vi "User Interface.vi"(10 "Test File Path":path=path "") -> ()   [LabVIEW 2020, in "Execution UI.lvclass"]
uses:
  Execution UI.lvclass
  Execution UI.lvclass/Execution UI.ctl
  Process/Process.lvclass
  <vilib>/Utility/miscctls.llb/LVNodeAndColumnTypeDef.ctl
  Private/TypeDefs/Execution State.ctl
  <vilib>/Platform/browser.llb/Open URL in Default Browser (string).vi
  Core/Result/Status.ctl
  Core/Result/Result.lvlib
  Result Model by Reference/Result Model by Reference.lvclass
  Core/Result/Type.ctl
  Core/Result/Result.ctl
  Configuration Manager/Configuration Manager.lvclass
  Support/Utilities.lvlib
  Error Handler/Error Handler.lvclass
  Framework/Test Finder/Test Finder.lvclass
  Framework/Test Runner/Test Runner.lvclass
  Result Model/Tree Item Filter.ctl
  Result Model/Result Model.lvclass
  Framework/Plugin/Plugin.lvclass
  C:/git/astemes-lunit/source/User Interface/Process/Process.lvclass
  C:/git/astemes-lunit/source/User Interface/Execution UI/Execution UI.lvclass
  C:/git/astemes-lunit/source/Framework/Result Observer/Result Observer.lvclass
panel:
  in  "Refresh":bool
  in  "Run Selected Tests":bool
  in  "Stop":bool
  in  "Run All Tests":bool
  in  "Eject":bool
  in  "Collapse":bool
  in  "Expand":bool
  out "Progress bar":dbl(slide) scale=0.0..100.0
  out "Results":i32(listbox)=-1
  in  "Test Results":string[](tree)
  out "Shift?":bool
  in  "Filter fails":bool
  out "Description":string
  out "Status":string
  # "1"
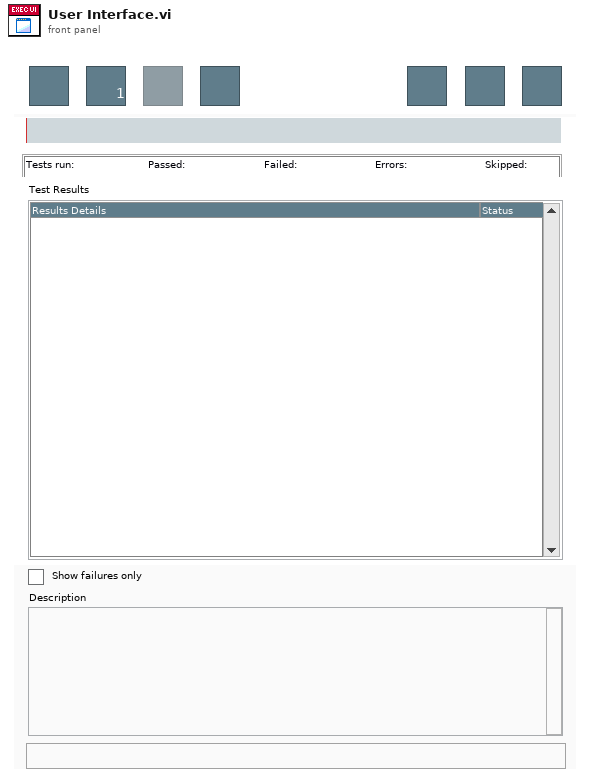
[diagram p1: front panel]
types:
  T1 = typedef "Execution UI.lvclass/Execution State.ctl" = enum16{"Idle", "Running"}
  T2 = typedef "Result.lvlib/Result.ctl" = cluster{"Name":string, "Message":string, "Description":string, "Status":T3, "Result Type":T4, "Execution Time":dbl}
  T3 = typedef "Result.lvlib/Status.ctl" = enum16{"", "Passed", "Failed", "Error", "Skipped", "Setup Error", "Broken", "Teardown Error"}
  T4 = typedef "Result.lvlib/Type.ctl" = enum16{"Test Case", "Test Suite", "Test Run", "Pass", "Fail", "Skip", "Pass if", "Fail if", "Pass if Error", "Fail if Error", "Pass if Equal", "Fail if Equal"}
  T5 = typedef "LVNodeAndColumnTypeDef.ctl" = cluster{"Node":string, "Column":i32}
  T6 = enum8{"Enabled", "Disabled", "Disabled and Grayed Out"}
  T7 = typedef "Result Model.lvclass/Tree Item Filter.ctl" = enum16{"All", "Only Fails", "Fails or else Not Executed"}
  T8 = enum32{"Invalid", "Standard", "Closed", "Hidden", "Minimized", "Maximized"}
  T9 = typedef "Result Model.lvclass/Statistics.ctl" = cluster{"Method Count":u32, "Executed Methods":u32, "Passed Methods":u32, "Failed Methods":u32, "Method Errors":u32, "Skipped Method":u32, "Progress [%]":dbl}
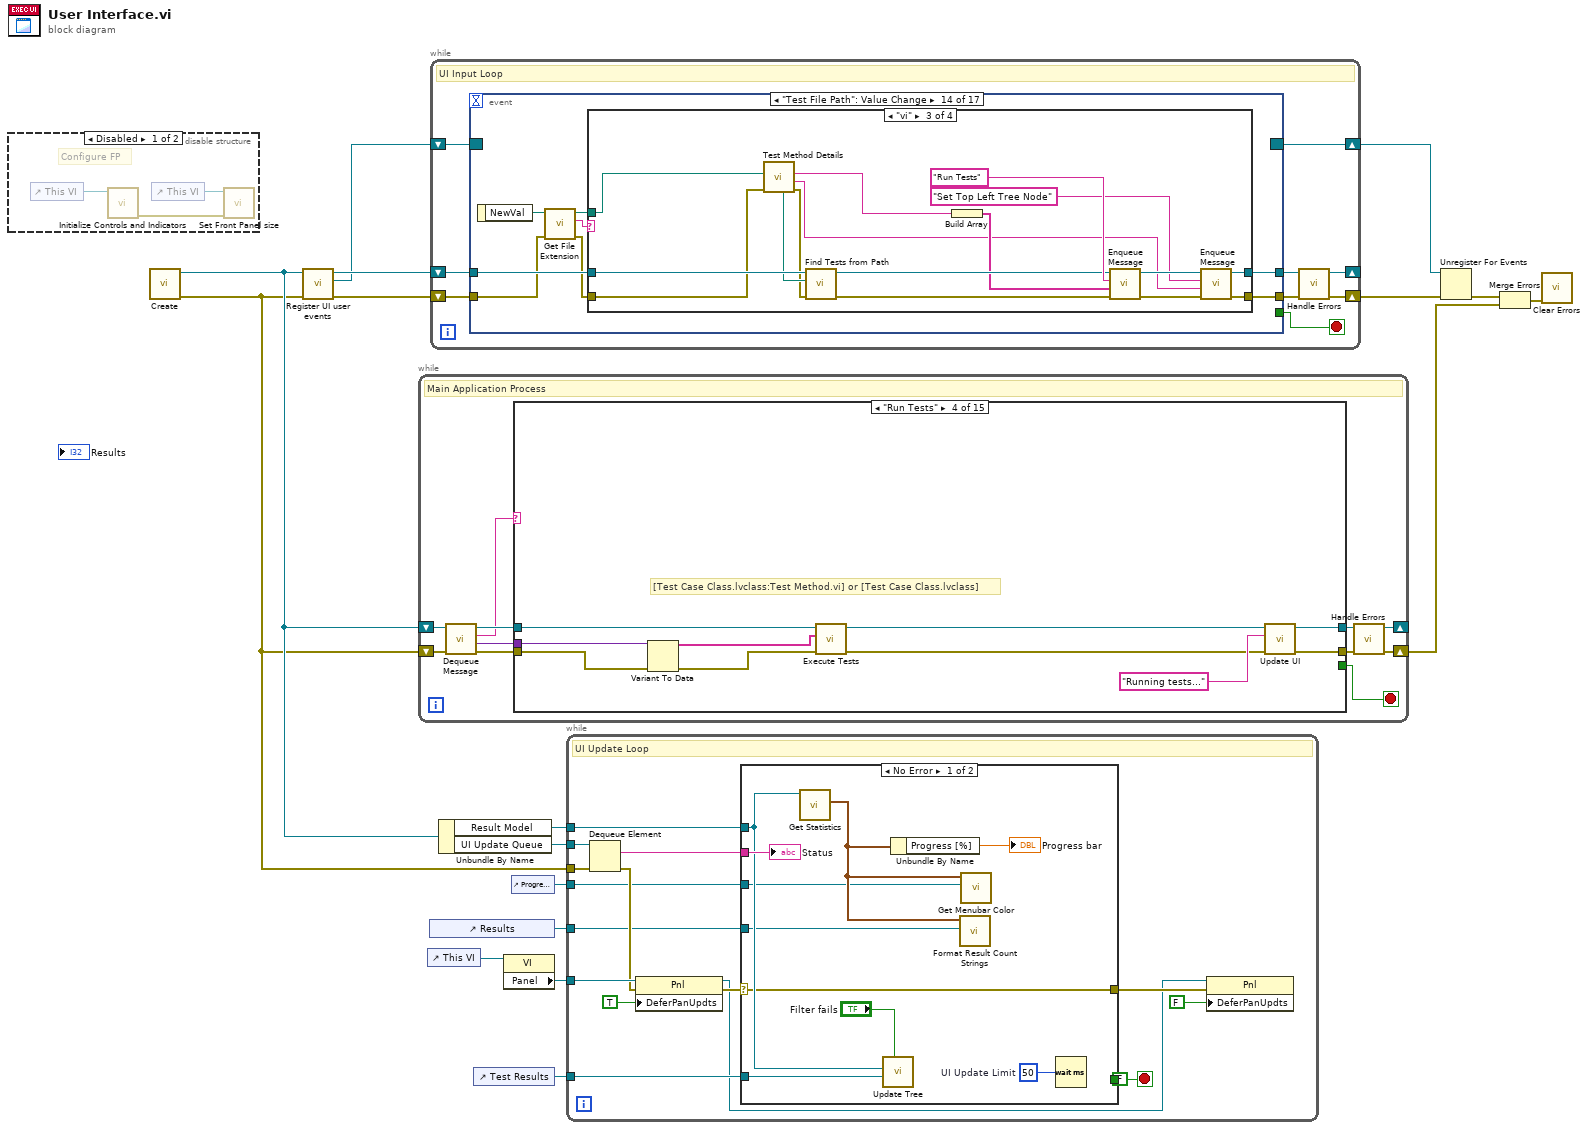
[diagram p0: block diagram]
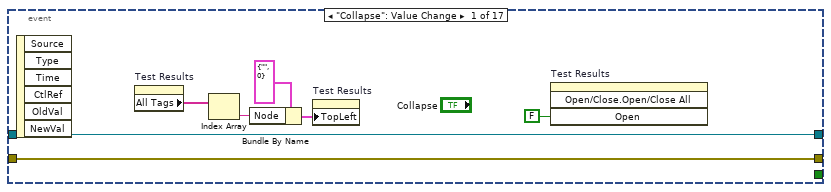
[diagram p2: hidden frame]
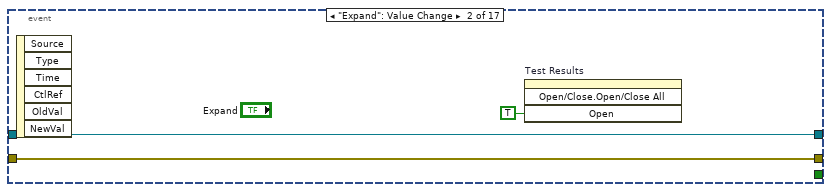
[diagram p3: hidden frame]
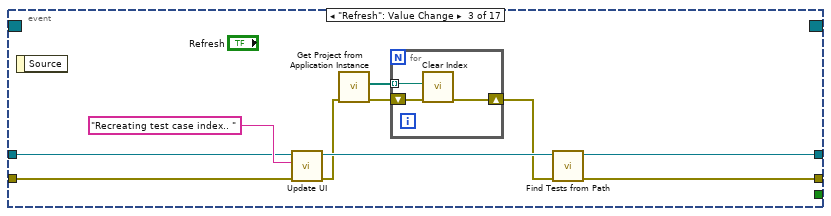
[diagram p4: hidden frame]
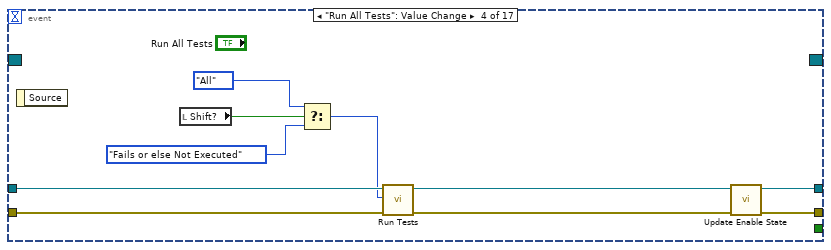
[diagram p5: hidden frame]
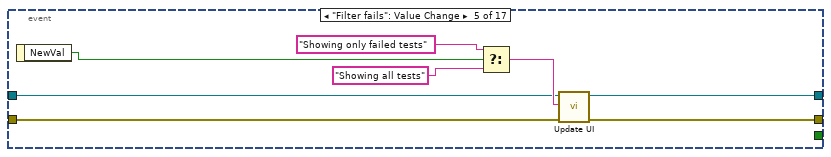
[diagram p6: hidden frame]
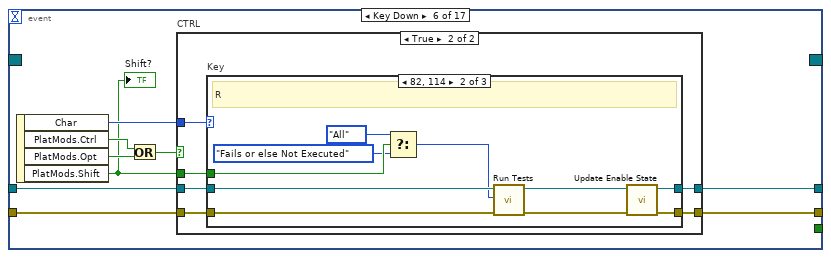
[diagram p7: hidden frame]
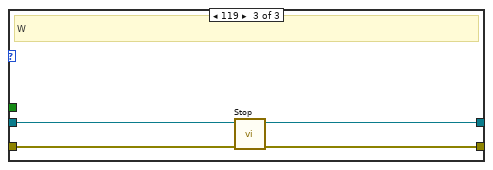
[diagram p10: hidden frame]
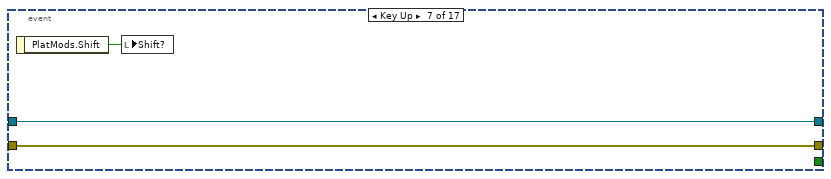
[diagram p11: hidden frame]
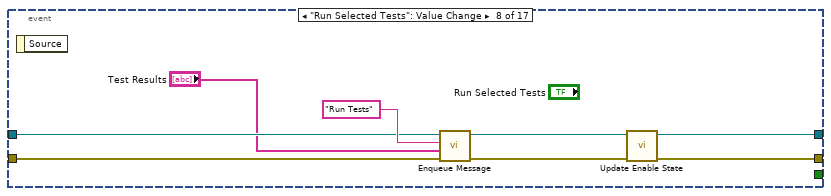
[diagram p12: hidden frame]
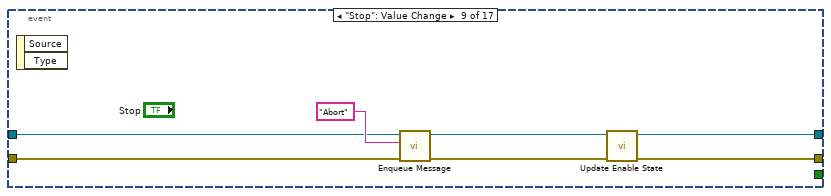
[diagram p13: hidden frame]
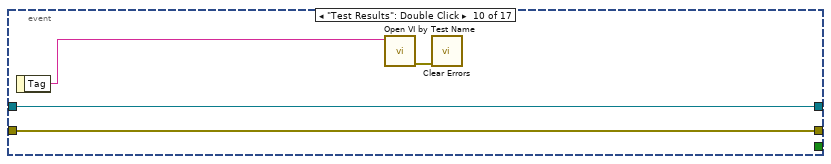
[diagram p14: hidden frame]
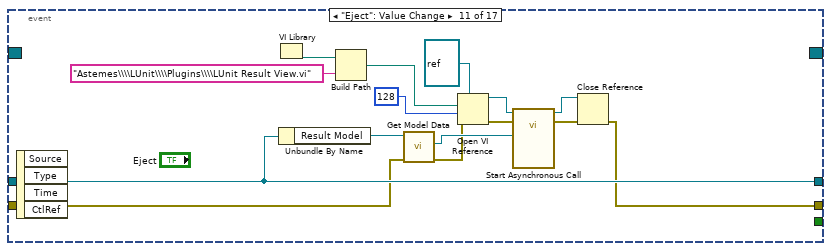
[diagram p15: hidden frame]
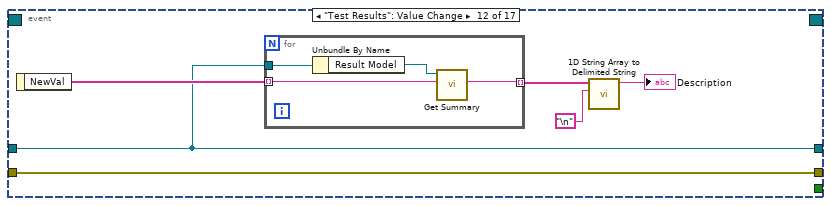
[diagram p16: hidden frame]
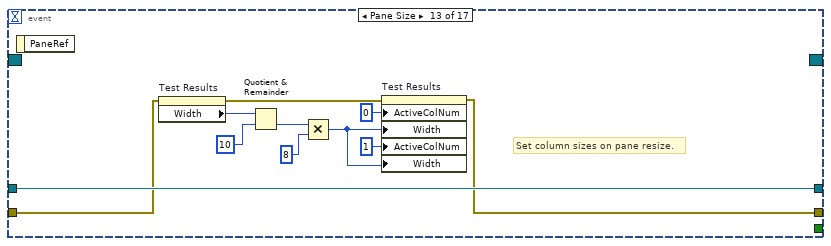
[diagram p17: hidden frame]
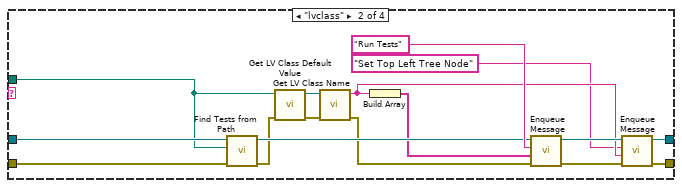
[diagram p19: hidden frame]
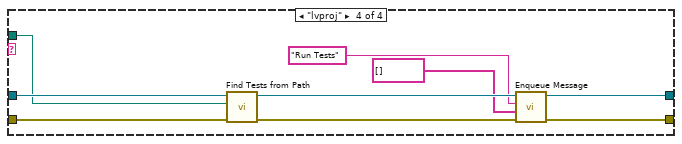
[diagram p20: hidden frame]
diagram:
  n1 = disable-structure shown="Disabled" {
    frame Disabled {
      # "Configure FP"
      n2 = control-ref of="This VI"() -> (w19:refnum<vi>)
      n3 = call "Initialize Controls and Indicators.vi"("VI in"=w19) -> ("error out"=w18:errorcluster)  [unwired: 10 in]
      n4 = control-ref of="This VI"() -> (w20:refnum<vi>)
      n5 = call "Set Front Panel size.vi"("error in (no error)"=w18, "VI in"=w20) -> ()  [unwired: 9 in, 1 out]
    }
    frame Enabled {
    }
  }
  n6 = call "Create.vi"() -> ("error out"=w3:errorcluster, "Execution UI Out"=w9:refnum<class "Execution UI.lvclass">)  [unwired: 10 in]
  n7 = call "Register UI user events.vi"("error in (no error)"=w3, "Execution UI In"=w9) -> ("error out"=w16:errorcluster, "Event Registration Refnum"=w14:refnum<event-registration>, "Execution UI Out"=w17:refnum<class "Execution UI.lvclass">)  [unwired: 7 in]
  n8 = while {
    shift-right: [w21] -> w13
    shift-left: w3 -> [w29]
    shift-right: [w23] -> _
    shift-left: w9 -> [w30]
    stop <- w26 stop-if-true
    # "Main Application Process"
    n9 = call "Dequeue Message.vi"("error in (no error)"=w29, "Process In"=w30) -> ("error out"=w27:errorcluster, "Message Data"=w24:variant, "Message"=w25:string, "Process Out"=w28:refnum<class "Execution UI.lvclass">)  [unwired: 6 in]
    n10 = case shown="\"Run Tests\"" w25 {
      selector: w25 -> [w31 _ _ _ _ _ _ _ _ w165 w172 _ w208 _ _]
      tunnel: w28 -> [w32 w41 w74 w78 w87 w99 w118 w135 w143 w170 w174 w187 w212 w226 w248]
      tunnel: [w33 w45 w61 w84 w88 w97 w119 w135 w143 w164 w177 w194 w220 w234 refnum<class "Execution UI.lvclass"> refnum ("Execution UI Out")] -> w23
      tunnel: w27 -> [w34 w39 w68 w80 w92 w102 w127 w136 w144 w169 w181 w193 w219 w233 w250]
      tunnel: [w35 w44 w63 w83 w91 w95 w121 w132 w144 w158 w175 w195 w221 w235 w255] -> w22
      tunnel: [_ _ _ _ _ _ _ _ _ _ _ _ _ _ TRUE] -> w26
      tunnel: w24 -> [_ _ w71 w76 _ w100 w113 w134 _ w168 w180 w192 w218 w232 _]
      frame Default {
        n11 = call "Unknown Command.vi"("error in (no error)"=w34, "String"=w31, "Process In"=w32) -> ("error out"=w35:errorcluster, "Process Out"=w33:refnum<class "Execution UI.lvclass">)  [unwired: 7 in]
      }
      frame "Init" {
        n12 = Current VI's Menubar() -> (w42:refnum<k9>)
        n13 = call "Populate Run-Time Menu.vi"("error in (no error)"=w39, "Menu in"=w42, "Execution UI In"=w41) -> ("error out"=w40:errorcluster, "Execution UI Out"=w38:refnum<class "Execution UI.lvclass">)  [unwired: 7 in]
        n14 = call <vilib>:"Is Path and Not Empty.vi"("path"="Test File Path") -> ("Is Path and Not Empty?"=w36:bool)  [unwired: 4 in]
        n15 = case shown="False" w36 {
          tunnel: [w53 w60] -> w47
          tunnel: [w52 w59] -> w46
          tunnel: w40 -> [w49 w59]
          tunnel: w38 -> [w51 w60]
          frame False {
            n16 = call "Get Project from Application Instance.vi"("error in (no error)"=w49) -> ("error out"=w50:errorcluster, "Open Projects"=w48:path[])  [unwired: 9 in]
            n17 = for {
              shift-right: [w58] -> w53
              shift-left: w51 -> [w56]
              shift-right: [w57] -> w52
              shift-left: w50 -> [w55]
              tunnel: w48 -> [w54] mode=indexing
              n18 = call "Find Tests from Path.vi"("error in (no error)"=w55, "Test File Path"=w54, "Execution UI in"=w56) -> ("error out"=w57:errorcluster, "Execution UI out"=w58:refnum<class "Execution UI.lvclass">)  [unwired: 7 in]
            }
          }
          frame True {
          }
        }
        n19 = call "Update Enable State.vi"("error in (no error)"=w46, "Execution UI In"=w47) -> ("error out"=w44:errorcluster, "Execution UI Out"=w45:refnum<class "Execution UI.lvclass">)  [unwired: 8 in]
        n20 = property on="Results" class="MCListbox (strict)"("ItemNames"=string[][] [["Last run:", "0/0", "Passed:", "0", "Failed:", "0", "Errors:", "0", "Skipped:", "0"]] ("Result Texts")) -> ()  [unwired: 2 in, 2 out]
      }
      frame "Find Tests" {
        # "Error when calling from launcher because FP not opened."
        n21 = Variant To Data(error in=w68, type=path "" ("Not A Path Constant"), Variant=w71) -> (data=w69:path, error out=w67:errorcluster)
        n22 = call <vilib>:"Set Busy.vi"("error in (no error)"=w67) -> ("error out"=w73:errorcluster)  [unwired: 9 in, 1 out]
        n23 = call <vilib>:"Clear Errors.vi"("error in (no error)"=w73, "specific error code to clear (0: all)"=26) -> ("error out"=w66:errorcluster)  [unwired: 4 in, 1 out]
        n24 = call "Find Tests.vi"("error in (no error)"=w66, "Project or Class Path"=w69, "Execution UI In"=w74) -> ("error out"=w62:errorcluster, "Execution UI Out"=w61:refnum<class "Execution UI.lvclass">)  [unwired: 7 in]
        n25 = call <vilib>:"Unset Busy.vi"("error in (no error)"=w62) -> ("error out"=w72:errorcluster)  [unwired: 10 in]
        n26 = call <vilib>:"Clear Errors.vi"("error in (no error)"=w72, "specific error code to clear (0: all)"=26) -> ("error out"=w63:errorcluster)  [unwired: 4 in, 1 out]
      }
      frame "Run Tests" {
        # "[Test Case Class.lvclass:Test Method.vi] or [Test Case Class.lvclass]"
        n27 = Variant To Data(error in=w80, Variant=w76) -> (data=w75:string[], error out=w77:errorcluster)  [unwired: 1 in]
        n28 = call "Execute Tests.vi"("error in (no error)"=w77, "Tests"=w75, "Execution UI In"=w78) -> ("error out"=w81:errorcluster, "Execution UI Out"=w79:refnum<class "Execution UI.lvclass">)  [unwired: 7 in]
        n29 = call "Update UI.vi"("error in (no error)"=w81, "Status"="Running tests...", "Execution UI In"=w79) -> ("error out"=w83:errorcluster, "Execution UI Out"=w84:refnum<class "Execution UI.lvclass">)  [unwired: 7 in]
      }
      frame "Abort" {
        n30 = Unbundle By Name(w87) -> ("Test Runner"=w85:refnum<class "Test Runner.lvclass">)
        n31 = call-dynamic "Abort.vi"("error in (no error)"=w92, "Test Runner in"=w85) -> ("error out"=w86:errorcluster)  [unwired: 9 in]
        n32 = Bundle By Name(cluster=w87, "Execution State"=Execution_State."Idle") -> (w93:refnum<class "Execution UI.lvclass">)
        n33 = call "Update UI.vi"("error in (no error)"=w86, "Status"="Aborting tests", "Execution UI In"=w93) -> ("error out"=w91:errorcluster, "Execution UI Out"=w88:refnum<class "Execution UI.lvclass">)  [unwired: 7 in]
      }
      frame "Result" {
        n34 = Variant To Data(error in=w102, type=T2 {"Name"="", "Message"="", "Description"="", "Status"=enum."Passed", "Result Type"=enum."Test Suite", "Execution Time"=0.0} ("Result"), Variant=w100) -> (data=w94:T2, error out=w96:errorcluster)
        n35 = in-place {
          in-place-border: w94 -> [w104]
          n36 = in-place-cluster #1(w99) -> ("Result Model"=w103:refnum<class "Result Model by Reference.lvclass">, "Plugins"=w105:map{string, refnum<class "Plugin.lvclass">})
          n37 = call-dynamic "Result.vi"("Results"=w104, "Result Model by Reference In"=w103) -> ()  [unwired: 9 in, 1 out]
          n38 = for {
            tunnel: w105 -> [w108] mode=indexing
            tunnel: w104 -> [w107]
            n39 = Unbundle By Name(w108) -> ("Plugin"=w106:refnum<class "Plugin.lvclass">)
            n40 = call-dynamic "Result.vi"("Result"=w107, "Plugin In"=w106) -> ()  [unwired: 9 in, 1 out]
          }
          n41 = in-place-cluster #1("Result Model"=w103, "Plugins"=w105) -> (w98:refnum<class "Execution UI.lvclass">)
        }
        n42 = call "Update Status on Result.vi"("error in (no error)"=w96, "Result"=w94, "Execution UI V2 in"=w98) -> ("error out"=w95:errorcluster, "Execution UI V2 out"=w97:refnum<class "Execution UI.lvclass">)  [unwired: 7 in]
      }
      frame "Test Run Result" {
        n43 = Variant To Data(error in=w127, type=T2 {"Name"="", "Message"="", "Description"="", "Status"=enum."Passed", "Result Type"=enum."Test Suite", "Execution Time"=0.0} ("Result"), Variant=w113) -> (data=w111:T2, error out=w114:errorcluster)
        n44 = local read "Test Results"() -> (w122:string[])
        n45 = Bundle By Name(cluster=w118, "Execution State"=Execution_State."Idle") -> (w110:refnum<class "Execution UI.lvclass">)
        n46 = property on="Test Results" class="Tree (strict)"("Val(Sgnl)"=w122) -> ()  [unwired: 2 in, 2 out]
        n47 = Unbundle By Name(w118) -> ("Start Time"=w116:timestamp)
        n48 = Get Date/Time In Seconds() -> (seconds since 1Jan1904=w117:timestamp)
        n49 = Subtract(x=w117, y=w116) -> (x-y=w115:dbl)
        n50 = call "Update Plugin Test End Result.vi"("Result"=w111, "Execution UI in"=w110) -> ("Execution UI out"=w109:refnum<class "Execution UI.lvclass">)  [unwired: 9 in]
        n51 = Format Into String(format string="Finnished in %.2f seconds", w115) -> (resulting string=w124:string)  [unwired: 2 in, 1 out]
        n52 = call "Update UI.vi"("error in (no error)"=w114, "Status"=w124, "Execution UI In"=w109) -> ("error out"=w126:errorcluster, "Execution UI Out"=w120:refnum<class "Execution UI.lvclass">)  [unwired: 7 in]
        n53 = call "Update Enable State.vi"("error in (no error)"=w126, "Execution UI In"=w120) -> ("error out"=w121:errorcluster, "Execution UI Out"=w119:refnum<class "Execution UI.lvclass">)  [unwired: 8 in]
      }
      frame "Set Top Left Tree Node" {
        n54 = Variant To Data(error in=w136, type="", Variant=w134) -> (data=w128:string, error out=w132:errorcluster)
        n55 = control-ref of="Test Results"() -> (w131:refnum<vi>)
        n56 = Bundle By Name(cluster=T5 {"Node"="", "Column"=0} ("Top Left Visible Cell"), "Node"=w128) -> (w129:T5)
        n57 = property on="Property Node" class="Tree (strict)"(reference=w131, "TopLeft"=w129) -> ()  [unwired: 1 in, 2 out]
      }
      frame "Update Enable State" {
        n58 = Unbundle By Name(w143) -> ("Execution State"=w142:T1)
        n59 = case shown="\"Running\"" w142 {
          tunnel: [T6."Enabled" ("Disabled") T6."Disabled and Grayed Out" ("Disabled")] -> w141
          tunnel: [T6."Disabled and Grayed Out" ("Disabled") T6."Enabled" ("Disabled")] -> w140
          tunnel: [T6."Disabled and Grayed Out" ("Disabled") T6."Enabled" ("Disabled")] -> w139
          tunnel: [T6."Disabled and Grayed Out" ("Disabled") T6."Enabled" ("Disabled")] -> w138
          tunnel: [T6."Disabled and Grayed Out" ("Disabled") T6."Enabled" ("Disabled")] -> w137
          frame "Running" {
          }
          frame "Idle" {
          }
        }
        n60 = property on="Stop" class="Bool"("DisabledEnum"=w141) -> ()  [unwired: 2 in, 2 out]
        n61 = property on="Run Selected Tests" class="Bool"("DisabledEnum"=w140) -> ()  [unwired: 2 in, 2 out]
        n62 = property on="Run All Tests" class="Bool"("DisabledEnum"=w139) -> ()  [unwired: 2 in, 2 out]
        n63 = property on="Refresh" class="Bool"("DisabledEnum"=w138) -> ()  [unwired: 2 in, 2 out]
        n64 = property on="Eject" class="Bool"("DisabledEnum"=w137) -> ()  [unwired: 2 in, 2 out]
      }
      frame "Ignore Dashed Tests" {
        n65 = Variant To Data(error in=w169, type=FALSE, Variant=w168) -> (data=w155:bool, error out=w159:errorcluster)
        n66 = Current VI's Menubar() -> (w166:refnum<k9>)
        n67 = Set Menu Item Info(6:w155, 7:w165, 11:w166) -> ()  [unwired: 4 in, 2 out]
        n68 = Bundle By Name(cluster=w170, "Ignore Dashed Tests?"=w155) -> (w164:refnum<class "Execution UI.lvclass">)
        n69 = call "Get Config File Path.vi"("error in (no error)"=w159) -> ("error out"=w161:errorcluster, "Config Directory"=w160:path)  [unwired: 9 in]
        n70 = call "Create.vi"("error in (no error)"=w161, "configuration file path"=w160) -> ("error out"=w156:errorcluster, "Configuration Manager out"=w157:refnum<class "Configuration Manager.lvclass">)  [unwired: 8 in]
        n71 = call "Set Dashed Tests Ignored.vi"("error in (no error)"=w156, "Ingore Dashed?"=w155, "Configuration Manager In"=w157) -> ("error out"=w162:errorcluster, "Configuration Manager Out"=w163:refnum<class "Configuration Manager.lvclass">)  [unwired: 7 in]
        n72 = call "Destroy.vi"("error in (no error)"=w162, "Configuration Manager In"=w163) -> ("error out"=w158:errorcluster)  [unwired: 9 in]
      }
      frame "Run Tests in Parallel" {
        w173 = TRUE  # Persist?
        n73 = Variant To Data(error in=w181, type=FALSE, Variant=w180) -> (data=w171:bool, error out=w176:errorcluster)
        n74 = Current VI's Menubar() -> (w178:refnum<k9>)
        n75 = Set Menu Item Info(6:w171, 7:w172, 11:w178) -> ()  [unwired: 4 in, 2 out]
        n76 = call "Configure Parallel Execution.vi"("error in (no error)"=w176, "Persist?"=w173, "Enable Parallel Execution?"=w171, "Execution UI In"=w174) -> ("error out"=w175:errorcluster, "Execution UI Out"=w177:refnum<class "Execution UI.lvclass">)  [unwired: 6 in]
      }
      frame "Execution Profiler..." {
        n77 = Variant To Data(error in=w193, type=TRUE, Variant=w192) -> (data=w182:bool, error out=w186:errorcluster)
        n78 = Select(t="Run a test to generate an execution analysis." ("Status"), s=w182, f="Execution profiler disabled" ("Status")) -> (s? t:f=w188:string)
        n79 = case shown="False" w182 {
          tunnel: [w200 w202] -> w184
          tunnel: w187 -> [w199 w205]
          tunnel: w186 -> [w198 w204]
          tunnel: [w197 w203] -> w185
          tunnel: "Execution Profiler.lvclass" -> [w196 w201]
          frame False {
            n80 = call "Clear Plugin.vi"("error in (no error)"=w198, "Plugin"=w196, "Execution UI in"=w199) -> ("error out"=w197:errorcluster, "Execution UI out"=w200:refnum<class "Execution UI.lvclass">)  [unwired: 7 in]
          }
          frame True {
            n81 = call "Init Plugin.vi"("error in (no error)"=w204, "Plugin"=w201, "Execution UI in"=w205) -> ("error out"=w203:errorcluster, "Execution UI out"=w202:refnum<class "Execution UI.lvclass">)  [unwired: 7 in]
          }
        }
        n82 = call "Update UI.vi"("error in (no error)"=w185, "Status"=w188, "Execution UI In"=w184) -> ("error out"=w195:errorcluster, "Execution UI Out"=w194:refnum<class "Execution UI.lvclass">)  [unwired: 7 in]
      }
      frame "Reporting..." {
        n83 = Variant To Data(error in=w219, type=TRUE, Variant=w218) -> (data=w215:bool, error out=w210:errorcluster)
        n84 = Select(t="Run a test to generate a report." ("Status"), s=w215, f="Report generation disabled" ("Status")) -> (s? t:f=w213:string)
        n85 = Current VI's Menubar() -> (w207:refnum<k9>)
        n86 = call "Configure Reporting Dialog.vi"("error in (no error)"=w210, "Execution UI In"=w212) -> ("error out"=w209:errorcluster, "Reporting Enabled?"=w206:bool, "Execution UI Out"=w211:refnum<class "Execution UI.lvclass">)  [unwired: 7 in]
        n87 = Set Menu Item Info(6:w206, 7:w208, 11:w207) -> ()  [unwired: 4 in, 2 out]
        n88 = call "Update UI.vi"("error in (no error)"=w209, "Status"=w213, "Execution UI In"=w211) -> ("error out"=w221:errorcluster, "Execution UI Out"=w220:refnum<class "Execution UI.lvclass">)  [unwired: 7 in]
      }
      frame "Coverage Analyzer..." {
        n89 = Variant To Data(error in=w233, type=TRUE, Variant=w232) -> (data=w223:bool, error out=w225:errorcluster)
        n90 = Select(t="Run a test to generate coverage analysis..." ("Status"), s=w223, f="Coverage analyzer disabled." ("Status")) -> (s? t:f=w228:string)
        n91 = case shown="False" w223 {
          tunnel: [w240 w242] -> w227
          tunnel: w226 -> [w239 w245]
          tunnel: w225 -> [w238 w244]
          tunnel: [w237 w243] -> w224
          tunnel: "Coverage Analyzer.lvclass" -> [w236 w241]
          frame False {
            n92 = call "Clear Plugin.vi"("error in (no error)"=w238, "Plugin"=w236, "Execution UI in"=w239) -> ("error out"=w237:errorcluster, "Execution UI out"=w240:refnum<class "Execution UI.lvclass">)  [unwired: 7 in]
          }
          frame True {
            n93 = call "Init Plugin.vi"("error in (no error)"=w244, "Plugin"=w241, "Execution UI in"=w245) -> ("error out"=w243:errorcluster, "Execution UI out"=w242:refnum<class "Execution UI.lvclass">)  [unwired: 7 in]
          }
        }
        n94 = call "Update UI.vi"("error in (no error)"=w224, "Status"=w228, "Execution UI In"=w227) -> ("error out"=w235:errorcluster, "Execution UI Out"=w234:refnum<class "Execution UI.lvclass">)  [unwired: 7 in]
      }
      frame "Stop" {
        n95 = control-ref of="This VI"() -> (w253:refnum<vi>)
        n96 = invoke on="Invoke Node" class="VI" method="FP.Close"(reference=w253, error in=w250) -> (reference out=w251:refnum<vi>, error out=w252:errorcluster)  [unwired: 1 in, 1 out]
        n97 = Close Reference(reference=w251, error in (no error)=w252) -> (error out=w246:errorcluster)
        n98 = Unbundle By Name(w248) -> ("Test Runner"=w247:refnum<class "Test Runner.lvclass">)
        n99 = call-dynamic "Abort.vi"("Test Runner in"=w247) -> ()  [unwired: 10 in, 1 out]
        n100 = call-dynamic "Clear.vi"("error in (no error)"=w246, "Execution UI In"=w248) -> ("error out"=w255:errorcluster)  [unwired: 9 in]
      }
    }
    n101 = call "Handle Errors.vi"("error in (no error)"=w22) -> ("error out"=w21:errorcluster)  [unwired: 10 in]
  }
  n102 = control-ref of="This VI"() -> (w6:refnum<vi>)
  n103 = control-ref of="Results"() -> (w2:refnum<vi>)
  n104 = while {
    shift-right: [w256] -> w12
    shift-left: w16 -> [w262]
    shift-right: [w258] -> _
    shift-left: w17 -> [w263]
    shift-right: [w260] -> w15
    shift-left: w14 -> [w259]
    stop <- w261 stop-if-true
    # "UI Input Loop"
    n105 = event shown="[13] \"Test File Path\": Value Change" {
      selector: w259 -> [_ _ _ _ _ _ _ _ _ _ _ _ _ _ _ _ _]
      dyn-events: [_ _ _ _ _ _ _ _ _ _ _ _ _ _ _ _ _] -> w260
      timeout: _ -> [_ _ _ _ _ _ _ _ _ _ _ _ _ _ _ _ _]
      tunnel: w263 -> [w269 w272 w282 w292 w298 w312 w339 w345 w352 w359 w369 w375 w395 w403 w450 w547 w553]
      tunnel: w262 -> [w270 w273 w281 w291 w300 w313 w340 w347 w355 w358 w361 w380 w385 w396 w449 w548 w550]
      tunnel: [w270 w273 w280 w295 w301 w311 w340 w344 w351 w358 w368 w380 w386 w401 w448 w548 w551] -> w257
      tunnel: [w269 w272 w278 w293 w299 w310 w339 w342 w349 w359 w369 w375 w395 w400 w447 w547 w552] -> w258
      tunnel: [_ _ _ _ _ _ _ _ _ _ _ _ _ _ _ TRUE _] -> w261
      event "Collapse": Value Change {
        n106 = event-data() -> ()  [unwired: 1 in, 6 out]
        n107 = property on="Test Results" class="Tree (strict)"() -> ("All Tags"=w267:string[])  [unwired: 2 in, 2 out]
        n108 = Index Array(array=w267) -> (element=w264:string)  [unwired: 1 in]
        n109 = Bundle By Name(cluster=T5 {"Node"="", "Column"=0} ("Top Left Visible Cell"), "Node"=w264) -> (w265:T5)
        n110 = property on="Test Results" class="Tree (strict)"("TopLeft"=w265) -> ()  [unwired: 2 in, 2 out]
        n111 = invoke on="Test Results" class="Tree (strict)" method="Open/Close.Open/Close All"("Open"=FALSE ("Open?")) -> ()  [unwired: 3 in, 4 out]
      }
      event "Expand": Value Change {
        n112 = event-data() -> ()  [unwired: 1 in, 6 out]
        n113 = invoke on="Test Results" class="Tree (strict)" method="Open/Close.Open/Close All"("Open"=TRUE ("Open?")) -> ()  [unwired: 3 in, 4 out]
      }
      event "Refresh": Value Change {
        n114 = event-data() -> ()  [unwired: 1 in, 1 out]
        n115 = call "Update UI.vi"("error in (no error)"=w281, "Status"="Recreating test case index.. ", "Execution UI In"=w282) -> ("error out"=w276:errorcluster, "Execution UI Out"=w279:refnum<class "Execution UI.lvclass">)  [unwired: 7 in]
        n116 = call "Get Project from Application Instance.vi"("error in (no error)"=w276) -> ("error out"=w275:errorcluster, "Open Projects"=w274:path[])  [unwired: 9 in]
        n117 = for {
          shift-right: [w286] -> w277
          shift-left: w275 -> [w285]
          tunnel: w274 -> [w284] mode=indexing
          n118 = call "Clear Index.vi"("error in (no error)"=w285, "Project Path"=w284) -> ("error out"=w286:errorcluster)  [unwired: 9 in]
        }
        n119 = call "Find Tests from Path.vi"("error in (no error)"=w277, "Execution UI in"=w279) -> ("error out"=w280:errorcluster, "Execution UI out"=w278:refnum<class "Execution UI.lvclass">)  [unwired: 8 in]
      }
      event "Run All Tests": Value Change {
        n120 = event-data() -> ()  [unwired: 1 in, 1 out]
        n121 = local read "Shift?"() -> (w288:bool)
        n122 = Select(t=Tree_Item_Filter."All" ("Filter"), s=w288, f=Tree_Item_Filter."Fails or else Not Executed") -> (s? t:f=w289:T7)
        n123 = call "Run Tests.vi"("error in (no error)"=w291, "Filter"=w289, "Execution UI in"=w292) -> ("error out"=w296:errorcluster, "Execution UI out"=w294:refnum<class "Execution UI.lvclass">)  [unwired: 7 in]
        n124 = call "Update Enable State.vi"("error in (no error)"=w296, "Execution UI In"=w294) -> ("error out"=w295:errorcluster, "Execution UI Out"=w293:refnum<class "Execution UI.lvclass">)  [unwired: 8 in]
      }
      event "Filter fails": Value Change {
        n125 = event-data() -> ("NewVal"=w297:bool)  [unwired: 1 in]
        n126 = Select(t="Showing only failed tests", s=w297, f="Showing all tests") -> (s? t:f=w304:string)
        n127 = call "Update UI.vi"("error in (no error)"=w300, "Status"=w304, "Execution UI In"=w298) -> ("error out"=w301:errorcluster, "Execution UI Out"=w299:refnum<class "Execution UI.lvclass">)  [unwired: 7 in]
      }
      event Key Down {
        n128 = event-data() -> ("Char"=w306:i16, "PlatMods.Ctrl"=w309:bool, "PlatMods.Opt"=w308:bool, "PlatMods.Shift"=w305:bool)  [unwired: 1 in]
        "Shift?" <- w305
        n129 = Or(x=w309, y=w308) -> (x .or. y?=w307:bool)
        n130 = case "CTRL" shown="True" w307 {
          tunnel: w313 -> [w314 w321]
          tunnel: w312 -> [w315 w320]
          tunnel: [w314 w319] -> w311
          tunnel: [w315 w318] -> w310
          tunnel: w306 -> [_ w317]
          tunnel: w305 -> [_ w316]
          frame False {
          }
          frame True {
            n131 = case "Key" shown="82, 114" w317 {
              tunnel: w321 -> [w322 w330 w336]
              tunnel: w320 -> [w323 w331 w337]
              tunnel: [w322 w333 w334] -> w319
              tunnel: [w323 w332 w335] -> w318
              tunnel: w316 -> [_ w327 _]
              frame Default {
              }
              frame 82, 114 {
                # "R"
                n132 = Select(t=Tree_Item_Filter."All" ("Filter"), s=w327, f=Tree_Item_Filter."Fails or else Not Executed" ("Filter")) -> (s? t:f=w324:T7)
                n133 = call "Run Tests.vi"("error in (no error)"=w330, "Filter"=w324, "Execution UI in"=w331) -> ("error out"=w328:errorcluster, "Execution UI out"=w329:refnum<class "Execution UI.lvclass">)  [unwired: 7 in]
                n134 = call "Update Enable State.vi"("error in (no error)"=w328, "Execution UI In"=w329) -> ("error out"=w333:errorcluster, "Execution UI Out"=w332:refnum<class "Execution UI.lvclass">)  [unwired: 8 in]
              }
              frame 119 {
                # "W"
                n135 = call-dynamic "Stop.vi"("error in (no error)"=w336, "Execution UI In"=w337) -> ("error out"=w334:errorcluster, "Execution UI Out"=w335:refnum<class "Execution UI.lvclass">)  [unwired: 8 in]
              }
            }
          }
        }
      }
      event Key Up {
        n136 = event-data() -> ("PlatMods.Shift"=w338:bool)  [unwired: 1 in]
        n137 = local write "Shift?"(w338) -> ()
      }
      event "Run Selected Tests": Value Change {
        n138 = event-data() -> ()  [unwired: 1 in, 1 out]
        n139 = call "Enqueue Message.vi"("error in (no error)"=w347, "Message Data"="Test Results", "Message"="Run Tests", "Process In"=w345) -> ("error out"=w348:errorcluster, "Process Out"=w343:refnum<class "Execution UI.lvclass">)  [unwired: 6 in]
        n140 = call "Update Enable State.vi"("error in (no error)"=w348, "Execution UI In"=w343) -> ("error out"=w344:errorcluster, "Execution UI Out"=w342:refnum<class "Execution UI.lvclass">)  [unwired: 8 in]
      }
      event "Stop": Value Change {
        n141 = event-data() -> ()  [unwired: 1 in, 2 out]
        n142 = call "Enqueue Message.vi"("error in (no error)"=w355, "Message"="Abort", "Process In"=w352) -> ("error out"=w354:errorcluster, "Process Out"=w350:refnum<class "Execution UI.lvclass">)  [unwired: 7 in]
        n143 = call "Update Enable State.vi"("error in (no error)"=w354, "Execution UI In"=w350) -> ("error out"=w351:errorcluster, "Execution UI Out"=w349:refnum<class "Execution UI.lvclass">)  [unwired: 8 in]
      }
      event "Test Results": Double Click {
        n144 = event-data() -> ("Tag"=w357:string)  [unwired: 1 in]
        n145 = call "Open VI by Test Name.vi"("Tag"=w357) -> ("error in (no error) 2"=w356:errorcluster)  [unwired: 10 in]
        n146 = call <vilib>:"Clear Errors.vi"("error in (no error)"=w356) -> ()  [unwired: 5 in, 2 out]
      }
      event "Eject": Value Change {
        n147 = event-data() -> ()  [unwired: 1 in, 4 out]
        n148 = VI Library() -> (path=w366:path)
        n149 = Unbundle By Name(w369) -> ("Result Model"=w364:refnum<class "Result Model by Reference.lvclass">)
        n150 = Build Path(base path=w366, name or relative path="Astemes\\\\LUnit\\\\Plugins\\\\LUnit Result View.vi" ("Relative Path from 1 to 2")) -> (appended path=w365:path)
        n151 = call "Get Model Data.vi"("error in (no error)"=w361, "Result Model by Reference In"=w364) -> ("error out"=w362:errorcluster, "Model Data"=w363:refnum<class "Result Model.lvclass">)  [unwired: 8 in]
        n152 = Open VI Reference(type specifier VI Refnum (for type only)=refnum<vi> refnum, vi path=w365, options=128, error in (no error)=w362) -> (vi reference=w374:refnum<vi>, error out=w373:errorcluster)  [unwired: 2 in]
        n153 = call-by-ref "Start Asynchronous Call"(reference=w374, error in=w373, "Model Data"=w363) -> (reference out=w372:refnum<vi>, error out=w371:errorcluster)  [unwired: 11 in]
        n154 = Close Reference(reference=w372, error in (no error)=w371) -> (error out=w368:errorcluster)
      }
      event "Test Results": Value Change {
        n155 = event-data() -> ("NewVal"=w376:string[])  [unwired: 1 in]
        n156 = for {
          tunnel: w375 -> [w384]
          tunnel: w376 -> [w381] mode=indexing
          tunnel: [w382] -> w378 mode=indexing
          n157 = Unbundle By Name(w384) -> ("Result Model"=w383:refnum<class "Result Model by Reference.lvclass">)
          n158 = call "Get Summary.vi"("Item"=w381, "Result Model by Reference In"=w383) -> ("Summary"=w382:string)  [unwired: 8 in, 1 out]
        }
        n159 = call <vilib>:"1D String Array to Delimited String.vi"("delimiter"="\n", "string array"=w378) -> ("delimited string"=→"Description":string)  [unwired: 9 in]
      }
      event Pane Size {
        # "Set column sizes on pane resize."
        n160 = event-data() -> ()  [unwired: 1 in, 1 out]
        n161 = property on="Test Results" class="Tree (strict)"(error in=w385) -> (error out=w387:errorcluster, "Width"=w388:u32)  [unwired: 1 in, 1 out]
        n162 = Quotient & Remainder(x=w388, y=u32 10) -> (floor(x/y)=w392:u32)  [unwired: 1 out]
        n163 = Multiply(x=w392, y=u32 8) -> (x*y=w389:u32)
        n164 = property on="Test Results" class="Tree (strict)"(error in=w387, "ActiveColNum"=0 ("Active Cell:Active Column Number"), "Width"=w389, "ActiveColNum"=1 ("Active Cell:Active Column Number"), "Width"=w389) -> (error out=w386:errorcluster)  [unwired: 1 in, 1 out]
      }
      event "Test File Path": Value Change {
        n165 = event-data() -> ("NewVal"=w402:path)  [unwired: 1 in]
        n166 = call <vilib>:"Get File Extension.vi"("error in (no error)"=w396, "file"=w402) -> ("error out"=w397:errorcluster, "lowercase file extension"=w398:string, "dup file"=w399:path)  [unwired: 5 in, 2 out]
        n167 = case shown="\"vi\"" w398 {
          tunnel: w403 -> [w405 w421 w437 w446]
          tunnel: w397 -> [w404 w420 w425 w445]
          tunnel: w399 -> [_ w416 w427 w444]
          tunnel: [w404 w411 w432 w441] -> w401
          tunnel: [w405 w409 w430 w440] -> w400
          frame Default {
          }
          frame "lvclass" {
            n168 = call "Find Tests from Path.vi"("error in (no error)"=w420, "Test File Path"=w416, "Execution UI in"=w421) -> ("error out"=w414:errorcluster, "Execution UI out"=w415:refnum<class "Execution UI.lvclass">)  [unwired: 7 in]
            n169 = call <vilib>:"Get LV Class Default Value.vi"("error in (no error)"=w414, "class path"=w416) -> ("error out"=w418:errorcluster, "object"=w417:refnum<class>)  [unwired: 8 in]
            n170 = call <vilib>:"Get LV Class Name.vi"("error in (no error)"=w418, "object"=w417) -> ("error out"=w413:errorcluster, "class name"=w408:string)  [unwired: 8 in]
            n171 = Build Array(w408) -> (w406:string[])
            n172 = call "Enqueue Message.vi"("error in (no error)"=w413, "Message Data"=w406, "Message"="Run Tests", "Process In"=w415) -> ("error out"=w412:errorcluster, "Process Out"=w410:refnum<class "Execution UI.lvclass">)  [unwired: 6 in]
            n173 = call "Enqueue Message.vi"("error in (no error)"=w412, "Message Data"=w408, "Message"="Set Top Left Tree Node", "Process In"=w410) -> ("error out"=w411:errorcluster, "Process Out"=w409:refnum<class "Execution UI.lvclass">)  [unwired: 6 in]
          }
          frame "vi" {
            n174 = call "Test Method Details.vi"("error in (no error)"=w425, "vi path"=w427) -> ("error out"=w424:errorcluster, "Test Case Class"=w422:string, "Test Method"=w423:string, "Test Case Path"=w426:path)  [unwired: 6 in]
            n175 = call "Find Tests from Path.vi"("error in (no error)"=w424, "Test File Path"=w426, "Execution UI in"=w437) -> ("error out"=w434:errorcluster, "Execution UI out"=w435:refnum<class "Execution UI.lvclass">)  [unwired: 7 in]
            n176 = Build Array(w423) -> (w428:string[])
            n177 = call "Enqueue Message.vi"("error in (no error)"=w434, "Message Data"=w428, "Message"="Run Tests", "Process In"=w435) -> ("error out"=w433:errorcluster, "Process Out"=w431:refnum<class "Execution UI.lvclass">)  [unwired: 6 in]
            n178 = call "Enqueue Message.vi"("error in (no error)"=w433, "Message Data"=w422, "Message"="Set Top Left Tree Node", "Process In"=w431) -> ("error out"=w432:errorcluster, "Process Out"=w430:refnum<class "Execution UI.lvclass">)  [unwired: 6 in]
          }
          frame "lvproj" {
            n179 = call "Find Tests from Path.vi"("error in (no error)"=w445, "Test File Path"=w444, "Execution UI in"=w446) -> ("error out"=w442:errorcluster, "Execution UI out"=w443:refnum<class "Execution UI.lvclass">)  [unwired: 7 in]
            n180 = call "Enqueue Message.vi"("error in (no error)"=w442, "Message Data"=string[] [] ("data"), "Message"="Run Tests", "Process In"=w443) -> ("error out"=w441:errorcluster, "Process Out"=w440:refnum<class "Execution UI.lvclass">)  [unwired: 6 in]
          }
        }
      }
      event Menu Selection (User) {
        n181 = event-data() -> ("ItemTag"=w451:string)  [unwired: 1 in]
        n182 = case shown="\"Reporting...\"" w451 {
          selector: w451 -> [_ _ _ w476 _ w505 w512 w518 _ _ _ _ _ _]
          tunnel: w450 -> [w465 w467 w474 w482 w490 w507 w514 w520 w525 w532 w536 w540 w541 w546]
          tunnel: w449 -> [w452 w466 w471 w480 w491 w506 w516 w522 w527 w529 w533 w537 w542 w545]
          tunnel: [w453 w466 w469 w478 w492 w504 w515 w521 w526 w530 w534 w538 w542 w544] -> w448
          tunnel: [w465 w467 w470 w479 w493 w503 w513 w519 w525 w532 w536 w540 w541 w543] -> w447
          frame "Full size" {
            n183 = control-ref of="This VI"() -> (w464:refnum<vi>)
            n184 = property on="Property Node" class="VI"(reference=w464, error in=w452, "FP.State"=T8."Maximized" ("Front Panel Window:State")) -> (error out=w455:errorcluster)  [unwired: 1 out]
            n185 = property on="Test Results" class="Tree (strict)"(error in=w455) -> (error out=w454:errorcluster, "Width"=w462:u32)  [unwired: 1 in, 1 out]
            n186 = Quotient & Remainder(x=w462, y=u32 10) -> (floor(x/y)=w461:u32)  [unwired: 1 out]
            n187 = Multiply(x=w461, y=u32 7) -> (x*y=w460:u32)
            n188 = property on="Test Results" class="Tree (strict)"(error in=w454, "ActiveColNum"=0 ("Active Cell:Active Column Number"), "Width"=w460, "ActiveColNum"=1 ("Active Cell:Active Column Number"), "Width"=w460) -> (error out=w453:errorcluster)  [unwired: 1 in, 1 out]
          }
          frame Default {
          }
          frame "Ignore Dashed Tests" {
            w473 = "Ignore Dashed Tests"
            n189 = Current VI's Menubar() -> (w475:refnum<k9>)
            n190 = Get Menu Item Info(7:w473, 11:w475) -> (4:w472:bool)  [unwired: 1 in, 6 out]
            n191 = Not(x=w472) -> (.not. x?=w468:bool)
            n192 = call "Enqueue Message.vi"("error in (no error)"=w471, "Message Data"=w468, "Message"=w473, "Process In"=w474) -> ("error out"=w469:errorcluster, "Process Out"=w470:refnum<class "Execution UI.lvclass">)  [unwired: 6 in]
          }
          frame "Run Tests in Parallel" {
            n193 = Current VI's Menubar() -> (w483:refnum<k9>)
            n194 = Get Menu Item Info(7:w476, 11:w483) -> (4:w481:bool)  [unwired: 1 in, 6 out]
            n195 = Not(x=w481) -> (.not. x?=w477:bool)
            n196 = call "Enqueue Message.vi"("error in (no error)"=w480, "Message Data"=w477, "Message"=w476, "Process In"=w482) -> ("error out"=w478:errorcluster, "Process Out"=w479:refnum<class "Execution UI.lvclass">)  [unwired: 6 in]
          }
          frame "Open Project or Test class" {
            n197 = call "File Dialog"("prompt"="Please select a test class or project file to load.", "pattern (all files)"="*.lvclass;*.lvproj;*.lvlib", "pattern label"="Project or class") -> ("selected path"=w489:path, "cancelled"=w485:bool, "error out"=w484:errorcluster)  [unwired: 9 in, 1 out]
            n198 = call <vilib>:"Clear Errors.vi"("error in (no error)"=w484) -> ()  [unwired: 5 in, 2 out]
            n199 = case shown="False" w485 {
              tunnel: [w495 w501] -> w493
              tunnel: [w494 w500] -> w492
              tunnel: w491 -> [w494 w499]
              tunnel: w490 -> [w495 w498]
              tunnel: w489 -> [_ w497]
              frame True {
              }
              frame False {
                n200 = call "Enqueue Message.vi"("error in (no error)"=w499, "Message Data"=w497, "Message"="Find Tests", "Process In"=w498) -> ("error out"=w500:errorcluster, "Process Out"=w501:refnum<class "Execution UI.lvclass">)  [unwired: 6 in]
              }
            }
          }
          frame "Reporting..." {
            n201 = Current VI's Menubar() -> (w502:refnum<k9>)
            n202 = Get Menu Item Info(7:w505, 8:w506, 11:w502) -> (0:w510:errorcluster, 4:w508:bool)  [unwired: 5 out]
            n203 = Not(x=w508) -> (.not. x?=w509:bool)
            n204 = call "Enqueue Message.vi"("error in (no error)"=w510, "Message Data"=w509, "Message"=w505, "Process In"=w507) -> ("error out"=w504:errorcluster, "Process Out"=w503:refnum<class "Execution UI.lvclass">)  [unwired: 6 in]
          }
          frame "Execution Profiler..." {
            n205 = Current VI's Menubar() -> (w511:refnum<k9>)
            n206 = call "Toggle Plugin.vi"("menu reference"=w511, "error in (no error)"=w516, "Item Tag"=w512, "Execution UI in"=w514) -> ("error out"=w515:errorcluster, "Execution UI out"=w513:refnum<class "Execution UI.lvclass">)  [unwired: 6 in]
          }
          frame "Coverage Analyzer..." {
            n207 = Current VI's Menubar() -> (w517:refnum<k9>)
            n208 = call "Toggle Plugin.vi"("menu reference"=w517, "error in (no error)"=w522, "Item Tag"=w518, "Execution UI in"=w520) -> ("error out"=w521:errorcluster, "Execution UI out"=w519:refnum<class "Execution UI.lvclass">)  [unwired: 6 in]
          }
          frame "Reset..." {
            n209 = control-ref of="This VI"() -> (w523:refnum<vi>)
            n210 = call "Initialize Controls and Indicators.vi"("error in (no error)"=w527, "VI in"=w523) -> ("error out"=w528:errorcluster)  [unwired: 9 in]
            n211 = control-ref of="This VI"() -> (w524:refnum<vi>)
            n212 = call "Set Front Panel size.vi"("error in (no error)"=w528, "VI in"=w524) -> ("error out"=w526:errorcluster)  [unwired: 9 in]
          }
          frame "Documentation..." {
            n213 = call-poly <vilib>:"Open URL in Default Browser.vi"("error in (no error)"=w529, "URL"="https://astemes.github.io/astemes-lunit/") -> ("error out"=w530:errorcluster)  [unwired: 4 in, 1 out]
          }
          frame "Report issue..." {
            n214 = call-poly <vilib>:"Open URL in Default Browser.vi"("error in (no error)"=w533, "URL"="https://github.com/astemes/astemes-lunit/issues") -> ("error out"=w534:errorcluster)  [unwired: 4 in, 1 out]
          }
          frame "Post an Idea..." {
            n215 = call-poly <vilib>:"Open URL in Default Browser.vi"("error in (no error)"=w537, "URL"="https://www.vipm.io/post/suggestion/?package_name=astemes_lib_lunit&return_url=/package/astemes_lib_lunit/") -> ("error out"=w538:errorcluster)  [unwired: 4 in, 1 out]
          }
          frame "About" {
            n216 = call "About Dialog.vi"() -> ()  [unwired: 12 in]
          }
          frame "Exit" {
            n217 = call-dynamic "Stop.vi"("error in (no error)"=w545, "Execution UI In"=w546) -> ("error out"=w544:errorcluster, "Execution UI Out"=w543:refnum<class "Execution UI.lvclass">)  [unwired: 8 in]
          }
        }
      }
      event User Event {
        n218 = event-data() -> ()  [unwired: 1 in, 4 out]
      }
      event Panel Close? {
        w554 = TRUE  # Discard?
        n219 = event-data() -> ()  [unwired: 1 in, 4 out]
        n220 = call-dynamic "Stop.vi"("error in (no error)"=w550, "Execution UI In"=w553) -> ("error out"=w551:errorcluster, "Execution UI Out"=w552:refnum<class "Execution UI.lvclass">)  [unwired: 8 in]
        n221 = event-data ("Event Filter Node")("Discard?"=w554) -> ()  [unwired: 1 in, 1 out]
      }
    }
    n222 = call "Handle Errors.vi"("error in (no error)"=w257) -> ("error out"=w256:errorcluster)  [unwired: 10 in]
  }
  n223 = Unbundle By Name(w9) -> ("Result Model"=w8:refnum<class "Result Model by Reference.lvclass">, "UI Update Queue"=w7:refnum<queue>)
  n224 = control-ref of="Test Results"() -> (w4:refnum<vi>)
  n225 = property on="Property Node" class="VI"(reference=w6) -> ("Panel"=w5:refnum<vi>)  [unwired: 1 in, 2 out]
  n226 = control-ref of="Progress bar"() -> (w1:refnum<vi>)
  n227 = while {
    tunnel: w3 -> [w568]
    tunnel: w8 -> [w567]
    tunnel: w7 -> [w566]
    tunnel: w5 -> [w564]
    tunnel: w4 -> [w558]
    tunnel: w2 -> [w556]
    tunnel: w1 -> [w555]
    stop <- w565 stop-if-true
    # "UI Update Loop"
    n228 = Dequeue Element(queue=w566, error in (no error)=w568) -> (element=w569:string, error out=w562:errorcluster)  [unwired: 1 in, 2 out]
    n229 = property on="Property Node" class="Pnl"(reference=w564, error in=w562, "DeferPanUpdts"=TRUE ("Defer Panel Updates")) -> (reference out=w557:refnum<vi>, error out=w561:errorcluster)
    n230 = case shown="No Error" w561 {
      selector: w561 -> [w574 w581]
      tunnel: w569 -> [w578 _]
      tunnel: w567 -> [w576 _]
      tunnel: [FALSE TRUE] -> w565
      tunnel: [w574 w581] -> w559
      tunnel: w558 -> [w572 _]
      tunnel: w556 -> [w571 _]
      tunnel: w555 -> [w570 _]
      frame No Error {
        w573 = u32 50  # UI Update Limit
        n231 = call "Get Statistics.vi"("Result Model in"=w576) -> ("Results"=w580:T9)  [unwired: 9 in, 1 out]
        n232 = call "Update Tree.vi"("Filter Fails?"="Filter fails", "Test Tree"=w572, "Result Model"=w576) -> ()  [unwired: 8 in, 1 out]
        n233 = Unbundle By Name(w580) -> ("Progress [%]"=→"Progress bar":dbl)
        n234 = call "Format Result Count Strings.vi"(10:"Results"=w571, 11:"Results"=w580) -> ()  [unwired: 9 in, 1 out]
        n235 = call "Get Menubar Color.vi"("Progress bar Ref"=w570, "Results"=w580) -> ()  [unwired: 9 in, 1 out]
        n236 = Wait (ms)(milliseconds to wait=w573) -> ()  [unwired: 1 out]
        "Status" <- w578
      }
      frame Error {
      }
    }
    n237 = property on="Property Node" class="Pnl"(reference=w557, error in=w559, "DeferPanUpdts"=FALSE ("Defer Panel Updates")) -> ()  [unwired: 2 out]
  }
  n238 = Unregister For Events(event registration refnum=w15, error in=w12) -> (error out=w11:errorcluster)
  n239 = Merge Errors(w11, w13) -> (w10:errorcluster)
  n240 = call <vilib>:"Clear Errors.vi"("error in (no error)"=w10) -> ()  [unwired: 5 in, 2 out]
